vi "Image.Zoom and Center.vi"(11 "2D Pict Ref":refnum<vi>) -> (2 "error out":errorcluster, 3 "Zoom Factor":dbl)   [LabVIEW 2018]
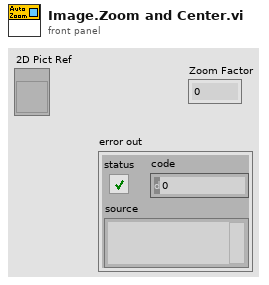
[diagram p1: front panel]
types:
  T1 = typedef "imagedata.ctl" = cluster{"image type":i32, "image depth":i32, "image":u8[], "mask":u8[], "colors":u32[], "Rectangle":cluster{"left":i16, "top":i16, "right":i16, "bottom":i16}}
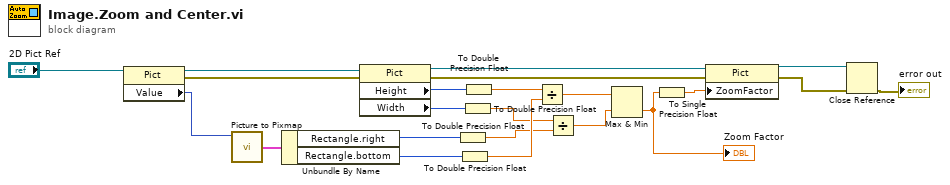
[diagram p0: block diagram]
diagram:
  n1 = property on="Property Node" class="Pict"(reference="2D Pict Ref") -> (reference out=w2:refnum<vi>, error out=w1:errorcluster, "Value"=w3:picture)  [unwired: 1 in]
  n2 = call <vilib>:"Picture to Pixmap.vi"("picture"=w3) -> ("image data"=w22:T1)  [unwired: 9 in, 1 out]
  n3 = Unbundle By Name(w22) -> ("Rectangle.right"=w21:i16, "Rectangle.bottom"=w20:i16)
  n4 = property on="Property Node" class="Pict"(reference=w2, error in=w1) -> (reference out=w11:refnum<vi>, error out=w8:errorcluster, "Height"=w19:u32, "Width"=w18:u32)
  n5 = To Double Precision Float(number=w21) -> (double precision float=w14:dbl)
  n6 = To Double Precision Float(number=w20) -> (double precision float=w16:dbl)
  n7 = To Double Precision Float(number=w18) -> (double precision float=w15:dbl)
  n8 = To Double Precision Float(number=w19) -> (double precision float=w17:dbl)
  n9 = Divide(x=w17, y=w16) -> (x/y=w13:dbl)
  n10 = Divide(x=w15, y=w14) -> (x/y=w12:dbl)
  n11 = Max & Min(x=w13, y=w12) -> (min(x,y)=w9:dbl)  [unwired: 1 out]
  "Zoom Factor" <- w9
  n12 = To Single Precision Float(number=w9) -> (single precision float=w10:sgl)
  n13 = property on="Property Node" class="Pict"(reference=w11, error in=w8, "ZoomFactor"=w10) -> (reference out=w7:refnum<vi>, error out=w6:errorcluster)
  n14 = Close Reference(reference=w7, error in (no error)=w6) -> (error out=→"error out":errorcluster)
